vi "String to Auto.vi"(11 "Auto Input":string) -> ()   [LabVIEW 2017]
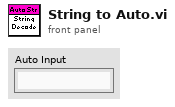
[diagram p1: front panel]
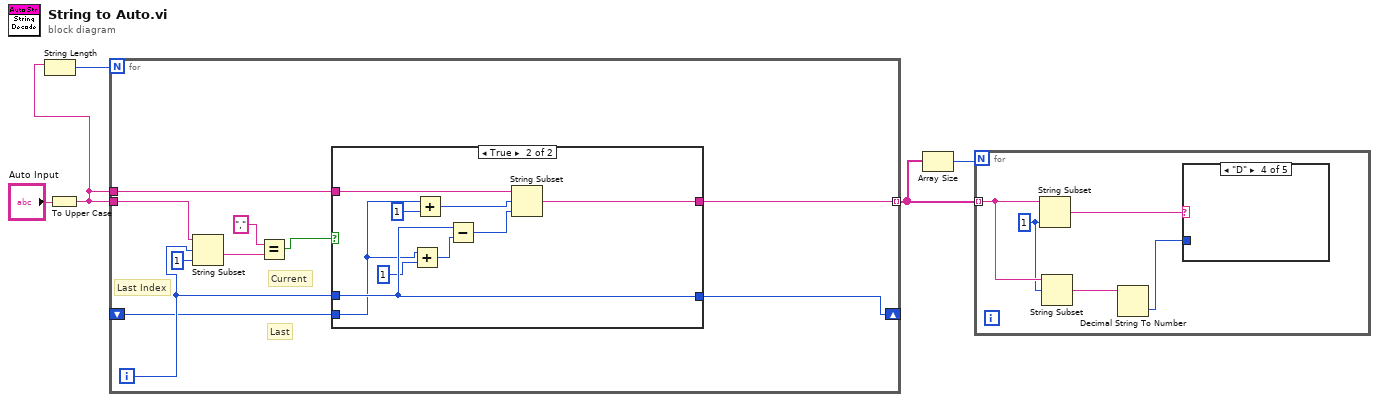
[diagram p0: block diagram]
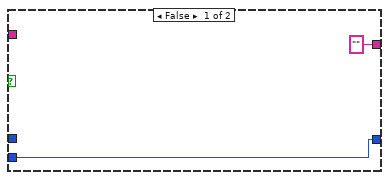
[diagram p6: hidden frame]
diagram:
  n1 = To Upper Case(1:"Auto Input") -> (0:w3:string)
  n2 = String Length(string=w3) -> (length=w5:i32)
  n3 = for {
    N: w5 -> [_]
    tunnel: w3 -> [w14]
    shift-right: [w8] -> _
    shift-left: _ -> [w7]
    tunnel: w3 -> [w11]
    tunnel: [w6] -> w1 mode=indexing
    i -> [w9]
    # "Last"
    # "Current"
    # "Last Index"
    n4 = String Subset(string=w14, offset (0)=w9, length (rest)=1 ("length (rest)")) -> (substring=w13:string)
    n5 = Equal?(x=",", y=w13) -> (x = y?=w10:bool)
    n6 = case shown="True" w10 {
      tunnel: w11 -> [_ w26]
      tunnel: w9 -> [_ w25]
      tunnel: [w17 w25] -> w8
      tunnel: w7 -> [w17 w21]
      tunnel: ["" w18] -> w6
      frame False {
      }
      frame True {
        n7 = Add(x=w21, y=1) -> (x+y=w19:i32)
        n8 = Add(x=w21, y=1) -> (x+y=w22:i32)
        n9 = Subtract(x=w25, y=w19) -> (x-y=w24:i32)
        n10 = String Subset(string=w26, offset (0)=w22, length (rest)=w24) -> (substring=w18:string)
      }
    }
  }
  n11 = Array Size(array=w1) -> (size(s)=w2:i32)
  n12 = for {
    N: w2 -> [_]
    tunnel: w1 -> [w30] mode=indexing
    w29 = 1 ("length (rest)")
    n13 = String Subset(string=w30, length (rest)=w29) -> (substring=w31:string)  [unwired: 1 in]
    n14 = String Subset(string=w30, offset (0)=w29) -> (substring=w28:string)  [unwired: 1 in]
    n15 = Decimal String To Number(string=w28) -> (number=w27:i32)  [unwired: 2 in, 1 out]
    n16 = case shown="\"D\"" w31 {
      tunnel: w27 -> [_ _ _ _ _]
      frame "B", Default {
      }
      frame "L" {
      }
      frame "R" {
      }
      frame "D" {
      }
      frame "F" {
      }
    }
  }
